vi "Graph_Server_Time_Get_Check (SubVI).vi"(8 "Error In":errorcluster, 11 "Boolean in":refnum<vi>) -> (0 "Error Out":errorcluster)   [LabVIEW 2018]
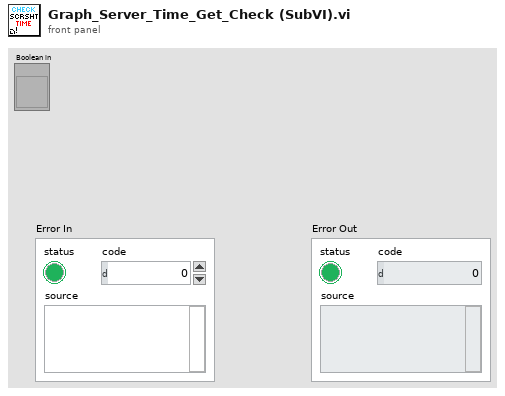
[diagram p1: front panel]
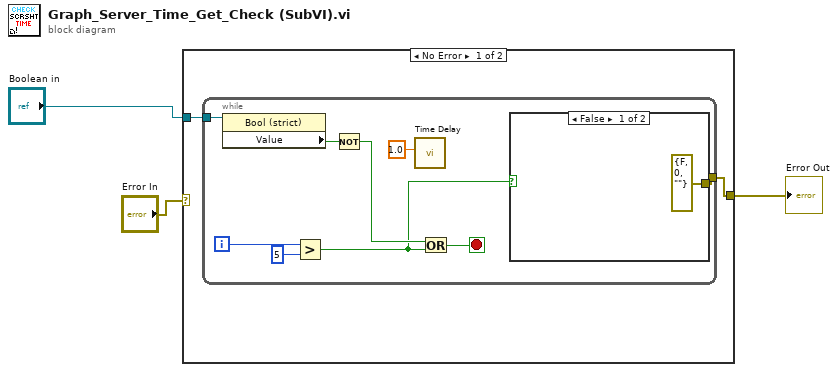
[diagram p0: block diagram]
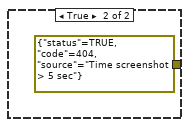
[diagram p2: hidden frame]
diagram:
  n1 = case shown="No Error" "Error In" {
    selector: "Error In" -> [_ w17]
    tunnel: "Boolean in" -> [w5 _]
    tunnel: [w4 w17] -> w1
    frame No Error {
      n2 = while {
        tunnel: [w8] -> w4
        tunnel: w5 -> [w6]
        i -> [w14]
        stop <- w11 stop-if-true
        n3 = property on="Property Node" class="Bool (strict)"(reference=w6) -> ("Value"=w7:bool)  [unwired: 1 in, 2 out]
        n4 = Greater?(x=w14, y=5) -> (0:w9:bool)
        n5 = Not(x=w7) -> (.not. x?=w12:bool)
        n6 = call "Time Delay"("Delay Time (s)"=1.0) -> ()  [unwired: 10 in, 1 out]
        n7 = Or(x=w12, y=w9) -> (x .or. y?=w11:bool)
        n8 = case shown="False" w9 {
          tunnel: [errorcluster {"status"=FALSE, "code"=0, "source"=""} ("Error Out") errorcluster {"status"=TRUE, "code"=404, "source"="Time screenshot > 5 sec"} ("Error Out")] -> w8
          frame False {
          }
          frame True {
          }
        }
      }
    }
    frame Error {
    }
  }
  "Error Out" <- w1
